vi "Check All Groups for Conflicts.vi"(8 "error in (no error)":errorcluster, 11 "Item Ref in":T1 format="%.0x") -> (0 "error out":errorcluster)   [LabVIEW 2020, in "Modbus Master System Explorer.lvlib"]
uses:
  Modbus Master System Explorer.lvlib
  <vilib>/NI VeriStand/Custom Device API/Custom Device Item Ref.ctl
  Shared/Constants.vi
  <vilib>/NI VeriStand/Custom Device Tools/Custom Device Utility Library/Custom Device Utility Library.lvlib
  Shared/Modbus Master Shared.lvlib
  <vilib>/NI VeriStand/Custom Device API/Custom Device API.lvlib
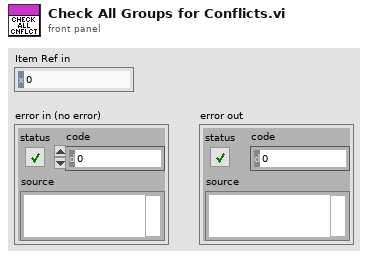
[diagram p1: front panel]
types:
  T1 = typedef "Custom Device API.lvlib/Custom Device Item Ref.ctl" = u64
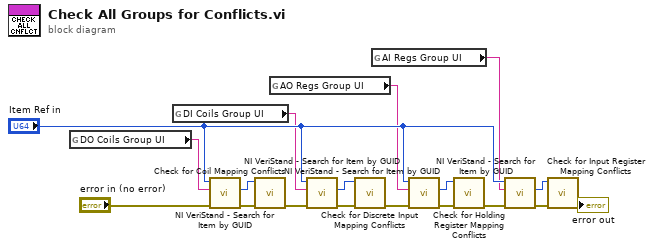
[diagram p0: block diagram]
diagram:
  n1 = global read "Constants.vi" "DO Coils Group UI"() -> (w1:string)
  n2 = global read "Constants.vi" "DI Coils Group UI"() -> (w5:string)
  n3 = call <vilib>:"NI VeriStand - Search for Item by GUID.vi"("error in"="error in (no error)", "Item GUID"=w1, "Section Ref in"="Item Ref in") -> ("error out"=w4:errorcluster, "Item Ref"=w2:T1)  [unwired: 5 in, 2 out]
  n4 = call "Check for Coil Mapping Conflicts.vi"("error in (no error)"=w4, "Coiil Group Ref in"=w2) -> ("error out"=w15:errorcluster)  [unwired: 6 in, 3 out]
  n5 = global read "Constants.vi" "AO Regs Group UI"() -> (w6:string)
  n6 = call <vilib>:"NI VeriStand - Search for Item by GUID.vi"("error in"=w15, "Item GUID"=w5, "Section Ref in"="Item Ref in") -> ("error out"=w12:errorcluster, "Item Ref"=w13:T1)  [unwired: 5 in, 2 out]
  n7 = call "Check for Discrete Input Mapping Conflicts.vi"("error in (no error)"=w12, "Coiil Group Ref in"=w13) -> ("error out"=w16:errorcluster)  [unwired: 6 in, 3 out]
  n8 = global read "Constants.vi" "AI Regs Group UI"() -> (w7:string)
  n9 = call <vilib>:"NI VeriStand - Search for Item by GUID.vi"("error in"=w16, "Item GUID"=w6, "Section Ref in"="Item Ref in") -> ("error out"=w10:errorcluster, "Item Ref"=w11:T1)  [unwired: 5 in, 2 out]
  n10 = call "Check for Holding Register Mapping Conflicts.vi"("error in (no error)"=w10, "Group Ref in"=w11) -> ("error out"=w17:errorcluster)  [unwired: 6 in, 3 out]
  n11 = call <vilib>:"NI VeriStand - Search for Item by GUID.vi"("error in"=w17, "Item GUID"=w7, "Section Ref in"="Item Ref in") -> ("error out"=w9:errorcluster, "Item Ref"=w8:T1)  [unwired: 5 in, 2 out]
  n12 = call "Check for Input Register Mapping Conflicts.vi"("error in (no error)"=w9, "Group Ref in"=w8) -> ("error out"=→"error out":errorcluster)  [unwired: 6 in, 3 out]
